vi "StressDist_long.vi"(7 "Corrigido":bool, 8 "Error In":errorcluster, 11 "main_FGV_data":T1={"pipe_properties"={"out_radius"=0.0, "in_radius"=0.0, "out_diameter"=0.0, "in_diameter"=0.0, "thickness"=0.0, "inertia"=0.0, "area"=0.0}, "DirPath"=path "L:/Documentos/00 SERVIÇOS/Tensão residual/Olapa 10-2017/Dados/Primeira Seção/Furos", "DirReport"=path "L:/Documentos/00 SERVIÇOS/Tensão residual/Olapa 10-2017/RelatóriosOlapa/Teste", "Points"=[], "ovalization_data"={"AngOval"=[0.0, 60.0, 120.0, 22.5, 45.0, 67.5, 90.0, 112.5, 135.0, 157.5, 180.0], "OvalDiam"=[324.25, 324.6, 324.55, 324.25, 324.55, 324.65, 324.6, 324.65, 324.55, 324.5, 324.4], "Plots"={"Ref"={"X"=[], "Y"=[]}, "Elipse"={"X"=[], "Y"=[]}, "Points"={"X"=[], "Y"=[]}}, "Ampliation"=100.0, "Results"={"MD"=0.0, "mD"=0.0, "Dmed"=0.0, "Oval"=0.0, "ang"=0.0, "X0"=0.0, "Y0"=0.0}}, "StressDist_data"={"Long"={"Plot"=[], "Fit"=[], "ColorMap"=[], "Data"=[], "peirce_data"={"Plot"=[], "Index removidos"=[]}}, "Circ"={"Plot"=[], "Fit"=[], "ColorMap"=[], "Data"=[], "peirce_data"={"Plot"=[], "Index removidos"=[]}}, "Shear"={"Plot"=[], "Fit"=[], "ColorMap"=[], "Data"=[], "peirce_data"={"Plot"=[], "Index removidos"=[]}}, "Equivalent"={"Plot"=[], "Fit"=[], "ColorMap"=[], "Data"=[], "peirce_data"={"Plot"=[], "Index removidos"=[]}}}, "pressure_data"={"Pressure"=[], "StressCircOval"=[], "StressCirc"=[], "StressLong"=[], "Plot"=[], "Angle"=[]}}) -> (0 "Error Out":errorcluster, 3 "main_FGV_data-out":T1={"pipe_properties"={"out_radius"=0.0, "in_radius"=0.0, "out_diameter"=0.0, "in_diameter"=0.0, "thickness"=0.0, "inertia"=0.0, "area"=0.0}, "DirPath"=path "L:/Documentos/00 SERVIÇOS/Tensão residual/Olapa 10-2017/Dados/Primeira Seção/Furos", "DirReport"=path "L:/Documentos/00 SERVIÇOS/Tensão residual/Olapa 10-2017/RelatóriosOlapa/Teste", "Points"=[], "ovalization_data"={"AngOval"=[0.0, 60.0, 120.0, 22.5, 45.0, 67.5, 90.0, 112.5, 135.0, 157.5, 180.0], "OvalDiam"=[324.25, 324.6, 324.55, 324.25, 324.55, 324.65, 324.6, 324.65, 324.55, 324.5, 324.4], "Plots"={"Ref"={"X"=[], "Y"=[]}, "Elipse"={"X"=[], "Y"=[]}, "Points"={"X"=[], "Y"=[]}}, "Ampliation"=100.0, "Results"={"MD"=0.0, "mD"=0.0, "Dmed"=0.0, "Oval"=0.0, "ang"=0.0, "X0"=0.0, "Y0"=0.0}}, "StressDist_data"={"Long"={"Plot"=[], "Fit"=[], "ColorMap"=[], "Data"=[], "peirce_data"={"Plot"=[], "Index removidos"=[]}}, "Circ"={"Plot"=[], "Fit"=[], "ColorMap"=[], "Data"=[], "peirce_data"={"Plot"=[], "Index removidos"=[]}}, "Shear"={"Plot"=[], "Fit"=[], "ColorMap"=[], "Data"=[], "peirce_data"={"Plot"=[], "Index removidos"=[]}}, "Equivalent"={"Plot"=[], "Fit"=[], "ColorMap"=[], "Data"=[], "peirce_data"={"Plot"=[], "Index removidos"=[]}}}, "pressure_data"={"Pressure"=[], "StressCircOval"=[], "StressCirc"=[], "StressLong"=[], "Plot"=[], "Angle"=[]}})   [LabVIEW 2016]
uses:
  MainFGV/main_FGV_data.ctl
  MainFGV/pipe_properties.ctl
  StressCalculations/point_data.ctl
  Ovalization/ovalization_data.ctl
  StressDist_data.ctl
  StressDist_single_data.ctl
  Peirce/peirce_data.ctl
  Pressure/pressure_data.ctl
  UserLibraries/AlgoritmoGenetico/TypeDefs/basic_config.ctl
  UserLibraries/AlgoritmoGenetico/TypeDefs/termination_data.ctl
  StressDist_types.ctl
  Report/report_mods.ctl
panel:
  out "LongStressCM":dbl[][](graph)
  out "LongStress":cluster{"X":dbl[], "Y":dbl[]}[](graph) caption="Ovalização"
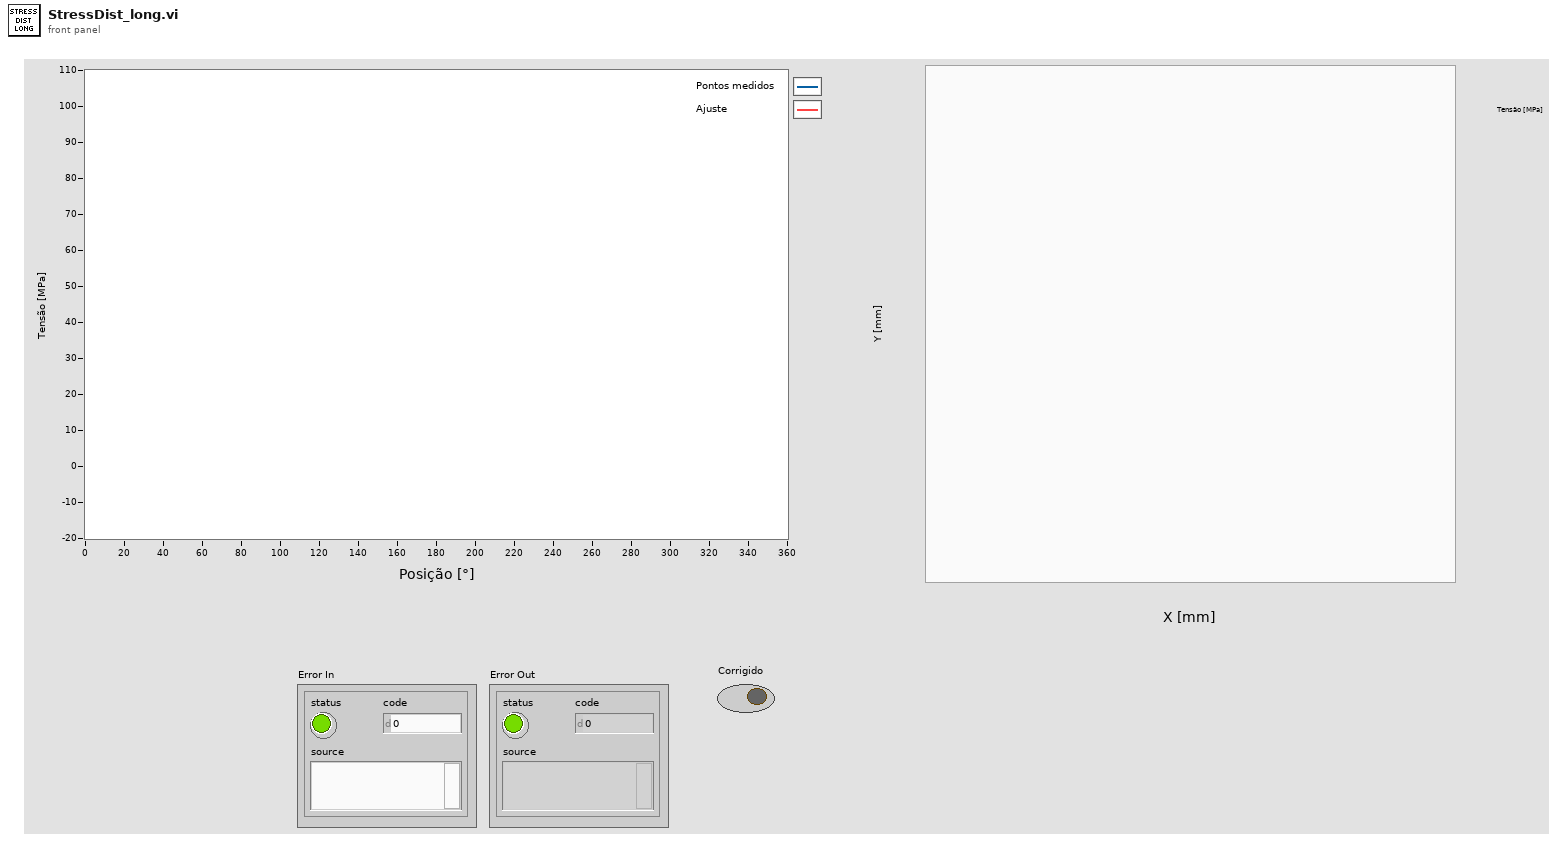
[diagram p1: front panel]
types:
  T1 = typedef "main_FGV_data.ctl" = cluster{"pipe_properties":T2, "DirPath":path, "DirReport":path, "Points":T3[], "ovalization_data":T4, "StressDist_data":T5, "pressure_data":T8}
  T2 = typedef "pipe_properties.ctl" = cluster{"out_radius":dbl, "in_radius":dbl, "out_diameter":dbl, "in_diameter":dbl, "thickness":dbl, "inertia":dbl, "area":dbl}
  T3 = typedef "point_data.ctl" = cluster{"LongStress":dbl, "CircStress":dbl, "ShearStress":dbl, "Pressure":dbl, "Angle":dbl, "Thickness":dbl, "HoleDiam":dbl, "EquiStress":dbl, "S1":dbl, "S2":dbl, "Beta":dbl}
  T4 = typedef "ovalization_data.ctl" = cluster{"AngOval":dbl[], "OvalDiam":dbl[], "Plots":cluster{"Ref":cluster{"X":dbl[], "Y":dbl[]}, "Elipse":cluster{"X":dbl[], "Y":dbl[]}, "Points":cluster{"X":dbl[], "Y":dbl[]}}, "Ampliation":dbl, "Results":cluster{"MD":dbl, "mD":dbl, "Dmed":dbl, "Oval":dbl, "ang":dbl, "X0":dbl, "Y0":dbl}}
  T5 = typedef "StressDist_data.ctl" = cluster{"Long":T6, "Circ":T6, "Shear":T6, "Equivalent":T6}
  T6 = typedef "StressDist_single_data.ctl" = cluster{"Plot":cluster{"Angle":dbl[], "Stress":dbl[]}[], "Fit":dbl[], "ColorMap":dbl[][], "Data":string[][], "peirce_data":T7}
  T7 = typedef "peirce_data.ctl" = cluster{"Plot":cluster{"Array":dbl[], "Array":dbl[]}[], "Index removidos":i32[]}
  T8 = typedef "pressure_data.ctl" = cluster{"Pressure":dbl[], "StressCircOval":dbl[], "StressCirc":dbl[], "StressLong":dbl[], "Plot":cluster{"Angle":dbl[], "Stress":dbl[]}[], "Angle":dbl[]}
  T9 = typedef "report_mods.ctl" = enum16{"Init", "Table", "Graph", "TablefromGraph", "End"}
  T10 = typedef "StressDist_types.ctl" = enum16{"Long", "Circ", "Shear", "Equivalent"}
  T11 = typedef "termination_data.ctl" = cluster{"MaxGen":cluster{"Generations":i32, "Active":bool}, "CostFunctionTol":cluster{"Tol":dbl, "Active":bool}, "GensEstab":cluster{"Generations":i32, "Active":bool}}
  T12 = typedef "basic_config.ctl" = cluster{"parameters_range":cluster{"Max":dbl, "Min":dbl}[], "Initial elements":i32}
  T13 = typedef "GenAlg_data.ctl" = cluster{"BasicCondfig":T12, "elements":T14[], "CostFunction":refnum<vi>, "GenerationData":T15, "SelectionData":T16, "SimulatedAnnealingData":T17, "CostFunctionData":variant, "MultiEval_data":T18, "TerminationData":T11}
  T14 = typedef "element.ctl" = cluster{"Parameters":dbl[], "Cost":dbl}
  T15 = typedef "geration_data.ctl" = cluster{"ElementsCreated":i32}
  T16 = typedef "selection_data.ctl" = cluster{"ElementsSelected":i32}
  T17 = typedef "SimulatedAnnealing_data.ctl" = cluster{"AnnealingFactor":dbl, "Active":bool}
  T18 = typedef "multi_eval_data.ctl" = cluster{"Active":bool, "MultiEvalFunction":refnum<vi>}
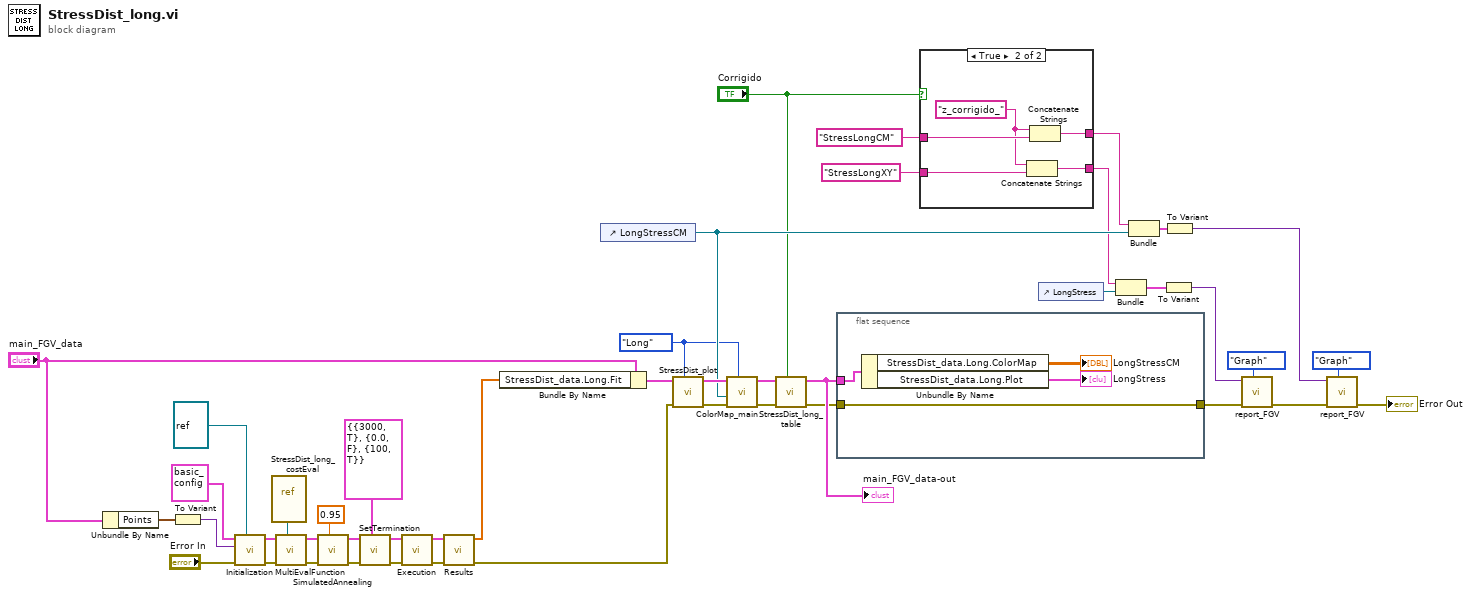
[diagram p0: block diagram]
diagram:
  w2 = StressDist_types."Long" ("StressDist_types")
  n1 = Unbundle By Name("main_FGV_data") -> ("Points"=w33:T3[])
  n2 = To Variant(anything=w33) -> (Variant=w32:variant)
  n3 = call "Initialization.vi"("CostFunction"=refnum<vi> refnum, "Error In"="Error In", "CostFunctionData"=w32, "basic_config"=T12 {"parameters_range"=[{"Max"=10000.0, "Min"=-10000.0}, {"Max"=10000.0, "Min"=-10000.0}, {"Max"=10000.0, "Min"=-10000.0}], "Initial elements"=20}) -> ("Error Out"=w44:errorcluster, "GenAlg_data"=w45:T13)  [unwired: 6 in]
  n4 = vi-ref "StressDist_long_costEval.vi"() -> (w28:refnum<vi>)
  n5 = call "MultiEvalFunction.vi"("MultiEvalFunction"=w28, "Error In"=w44, "GenAlg_data"=w45) -> ("Error Out"=w43:errorcluster, "GenAlg_data-out"=w39:T13)  [unwired: 7 in]
  n6 = call "SimulatedAnnealing.vi"("AnnealingFactor"=0.95, "Error In"=w43, "GenAlg_data"=w39) -> ("Error Out"=w42:errorcluster, "GenAlg_data-out"=w38:T13)  [unwired: 7 in]
  n7 = call "SetTermination.vi"("TerminationData"=T11 {"MaxGen"={"Generations"=3000, "Active"=TRUE}, "CostFunctionTol"={"Tol"=0.0, "Active"=FALSE}, "GensEstab"={"Generations"=100, "Active"=TRUE}}, "Error In"=w42, "GenAlg_data"=w38) -> ("Error Out"=w41:errorcluster, "GenAlg_data-out"=w37:T13)  [unwired: 7 in]
  n8 = call "Execution.vi"("Error In"=w41, "GenAlg_data"=w37) -> ("Error Out"=w40:errorcluster, "GenAlg_data-out"=w36:T13)  [unwired: 8 in]
  n9 = call "Results.vi"("Error In"=w40, "GenAlg_data"=w36) -> ("Error Out"=w27:errorcluster, "MinPoint"=w20:dbl[])  [unwired: 7 in, 1 out]
  n10 = Bundle By Name(cluster="main_FGV_data", "StressDist_data.Long.Fit"=w20) -> (w19:T1)
  n11 = control-ref of="LongStressCM"() -> (w11:refnum<vi>)
  n12 = call "StressDist_plot.vi"("StressDist_types"=w2, "Error In"=w27, "main_FGV_data"=w19) -> ("Error Out"=w18:errorcluster, "main_FGV_data-out"=w17:T1)  [unwired: 7 in]
  n13 = call "ColorMap_main.vi"("StressDist_types"=w2, "Error In"=w18, "RefCM"=w11, "main_FGV_data"=w17) -> ("Error Out"=w6:errorcluster, "main_FGV_data-out"=w4:T1)  [unwired: 6 in]
  n14 = call "StressDist_long_table.vi"("Corrigido"="Corrigido", "Error In"=w6, "main_FGV_data"=w4) -> ("Error Out"=w3:errorcluster, "main_FGV_data-out"=w5:T1)  [unwired: 7 in]
  "main_FGV_data-out" <- w5
  n15 = flat-sequence {
    tunnel: w5 -> [w49]
    tunnel: w3 -> [w47]
    tunnel: [w47] -> w25
    frame #0 {
      n16 = Unbundle By Name(w49) -> ("StressDist_data.Long.ColorMap"=→"LongStressCM":dbl[][], "StressDist_data.Long.Plot"=→"LongStress":cluster{"Angle":dbl[], "Stress":dbl[]}[])
    }
  }
  n17 = case shown="True" "Corrigido" {
    tunnel: "StressLongCM" -> [w51 w56]
    tunnel: "StressLongXY" -> [w50 w54]
    tunnel: [w51 w55] -> w8
    tunnel: [w50 w53] -> w7
    frame False {
    }
    frame True {
      w52 = "z_corrigido_" ("string")
      n18 = Concatenate Strings(w52, w54) -> (w53:string)
      n19 = Concatenate Strings(w52, w56) -> (w55:string)
    }
  }
  n20 = control-ref of="LongStress"() -> (w22:refnum<vi>)
  n21 = Bundle(w7, "LongStress"=w22) -> (w24:cluster{string, "LongStress":refnum<vi>})  [unwired: 1 in]
  n22 = Bundle(w8, "LongStressCM"=w11) -> (w13:cluster{string, "LongStressCM":refnum<vi>})  [unwired: 1 in]
  n23 = To Variant(anything=w24) -> (Variant=w23:variant)
  n24 = To Variant(anything=w13) -> (Variant=w12:variant)
  n25 = call "report_FGV.vi"("report_mods"=report_mods."Graph", "Error In"=w25, "Data in"=w23) -> ("Error Out"=w15:errorcluster)  [unwired: 8 in]
  n26 = call "report_FGV.vi"("report_mods"=report_mods."Graph", "Error In"=w15, "Data in"=w12) -> ("Error Out"=→"Error Out":errorcluster)  [unwired: 8 in]
